vi "set accessories settings.vi"(8 "error in (no error)":errorcluster, 10 "accessories_settings":T1, 11 "id":i32) -> (0 "error out":errorcluster, 3 "function return":i32)   [LabVIEW 2012, in "libximc.lvlib"]
doc: "result_t XIMC_API set_accessories_settings (device_t id, const accessories_settings_t* accessories_settings);"
uses:
  libximc.lvlib
  libximc.dll
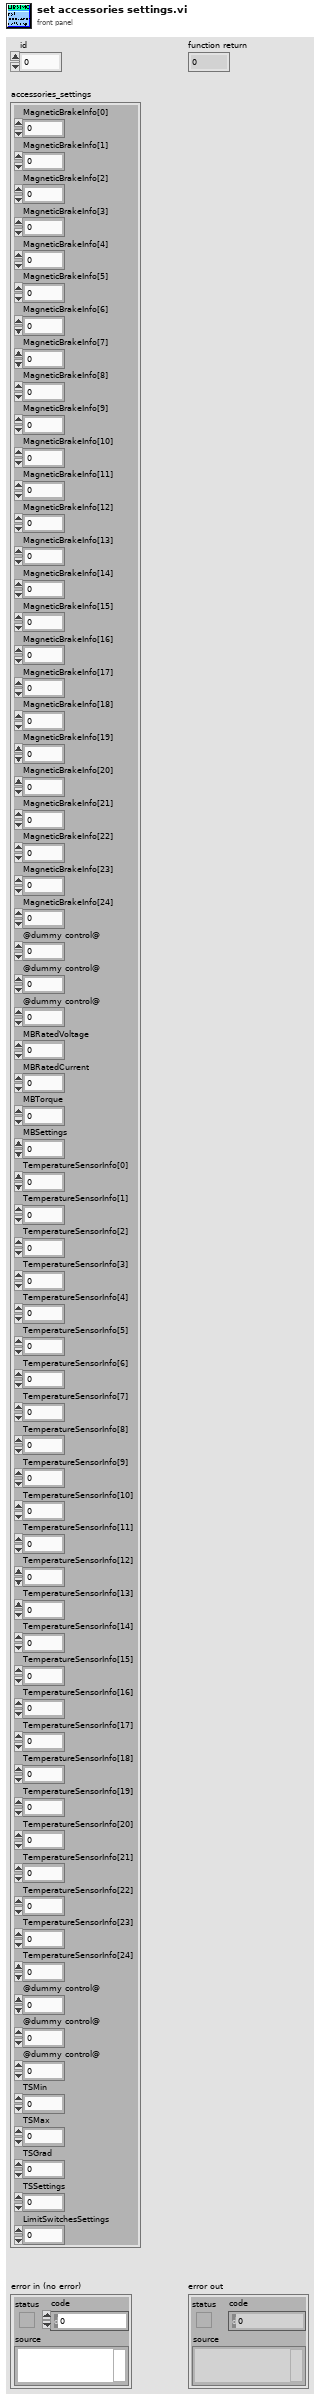
[diagram p1: front panel]
types:
  T1 = cluster{"MagneticBrakeInfo[0]":i8, "MagneticBrakeInfo[1]":i8, "MagneticBrakeInfo[2]":i8, "MagneticBrakeInfo[3]":i8, "MagneticBrakeInfo[4]":i8, "MagneticBrakeInfo[5]":i8, "MagneticBrakeInfo[6]":i8, "MagneticBrakeInfo[7]":i8, "MagneticBrakeInfo[8]":i8, "MagneticBrakeInfo[9]":i8, "MagneticBrakeInfo[10]":i8, "MagneticBrakeInfo[11]":i8, "MagneticBrakeInfo[12]":i8, "MagneticBrakeInfo[13]":i8, "MagneticBrakeInfo[14]":i8, "MagneticBrakeInfo[15]":i8, "MagneticBrakeInfo[16]":i8, "MagneticBrakeInfo[17]":i8, "MagneticBrakeInfo[18]":i8, "MagneticBrakeInfo[19]":i8, "MagneticBrakeInfo[20]":i8, "MagneticBrakeInfo[21]":i8, "MagneticBrakeInfo[22]":i8, "MagneticBrakeInfo[23]":i8, "MagneticBrakeInfo[24]":i8, "@dummy control@":i8, "@dummy control@":i8, "@dummy control@":i8, "MBRatedVoltage":sgl, "MBRatedCurrent":sgl, "MBTorque":sgl, "MBSettings":u32, "TemperatureSensorInfo[0]":i8, "TemperatureSensorInfo[1]":i8, "TemperatureSensorInfo[2]":i8, "TemperatureSensorInfo[3]":i8, "TemperatureSensorInfo[4]":i8, "TemperatureSensorInfo[5]":i8, "TemperatureSensorInfo[6]":i8, "TemperatureSensorInfo[7]":i8, "TemperatureSensorInfo[8]":i8, "TemperatureSensorInfo[9]":i8, "TemperatureSensorInfo[10]":i8, "TemperatureSensorInfo[11]":i8, "TemperatureSensorInfo[12]":i8, "TemperatureSensorInfo[13]":i8, "TemperatureSensorInfo[14]":i8, "TemperatureSensorInfo[15]":i8, "TemperatureSensorInfo[16]":i8, "TemperatureSensorInfo[17]":i8, "TemperatureSensorInfo[18]":i8, "TemperatureSensorInfo[19]":i8, "TemperatureSensorInfo[20]":i8, "TemperatureSensorInfo[21]":i8, "TemperatureSensorInfo[22]":i8, "TemperatureSensorInfo[23]":i8, "TemperatureSensorInfo[24]":i8, "@dummy control@":i8, "@dummy control@":i8, "@dummy control@":i8, "TSMin":sgl, "TSMax":sgl, "TSGrad":sgl, "TSSettings":u32, "LimitSwitchesSettings":u32}
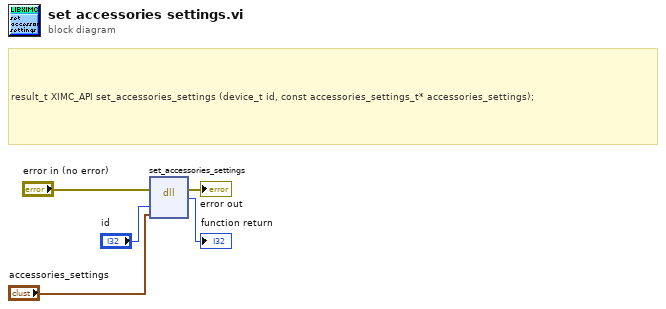
[diagram p0: block diagram]
diagram:
  # "result_t XIMC_API set_accessories_settings (device_t id, const accessories_settings_t* accessories_settings);"
  n1 = dll-call lib="C:/Users/Vasily/Att_examples/LabVIEW_example/libximc.*" fn="set_accessories_settings"(error in="error in (no error)", "id"="id", "accessories_settings"="accessories_settings") -> (error out=→"error out":errorcluster, →"function return":i32)  [unwired: 4 in, 1 out]
